vi "Task01.vi"() -> ()   [LabVIEW 2017]
panel:
  in  "Stop Button":bool
  in  "Switch01":bool
  out "LED07":bool
  out "LED08":bool
  out "LED06":bool
  out "LED05":bool
  out "LED04":bool
  out "LED03":bool
  out "LED02":bool
  out "LED01":bool
  in  "Switch08":bool
  in  "Switch07":bool
  in  "Switch06":bool
  in  "Switch05":bool
  in  "Switch04":bool
  in  "Switch03":bool
  in  "Switch02":bool
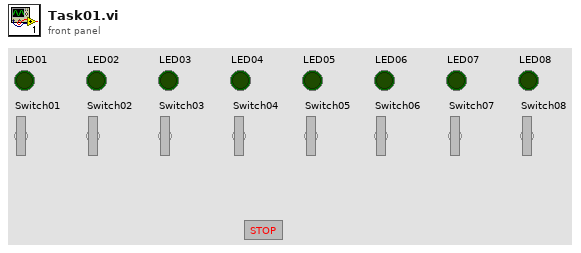
[diagram p1: front panel]
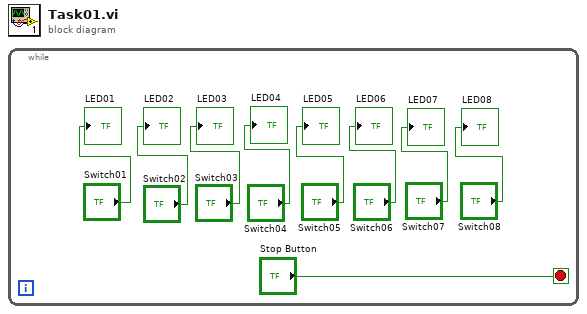
[diagram p0: block diagram]
diagram:
  n1 = while {
    stop <- "Stop Button" stop-if-true
    "LED01" <- "Switch01"
    "LED02" <- "Switch02"
    "LED03" <- "Switch03"
    "LED04" <- "Switch04"
    "LED05" <- "Switch05"
    "LED06" <- "Switch06"
    "LED08" <- "Switch08"
    "LED07" <- "Switch07"
  }
